vi "uti_IsInSubPanel.vi"(8 "error in (no error)":errorcluster, 11 "UI_Actor in":refnum<class "UI_Actor.lvclass">) -> (0 "error out":errorcluster, 2 "Running in SubPanel?":bool, 3 "UI_Actor out":refnum<class "UI_Actor.lvclass">)   [LabVIEW 2020, in "UI_Actor.lvlib" / "UI_Actor.lvclass"]
uses:
  UI_Actor.lvclass
  UI_Actor.lvclass/UI_Actor.ctl
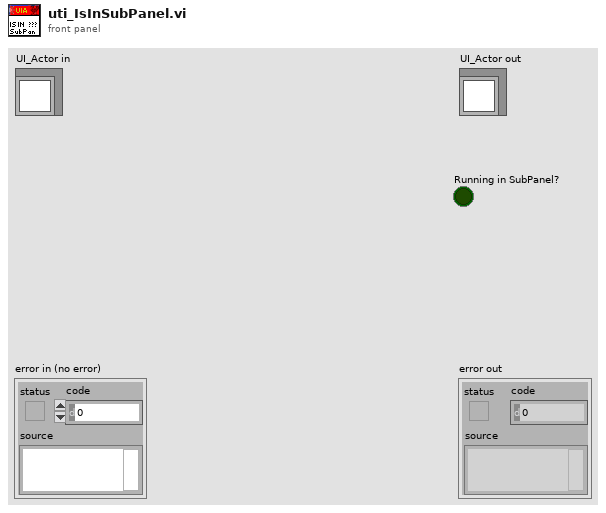
[diagram p1: front panel]
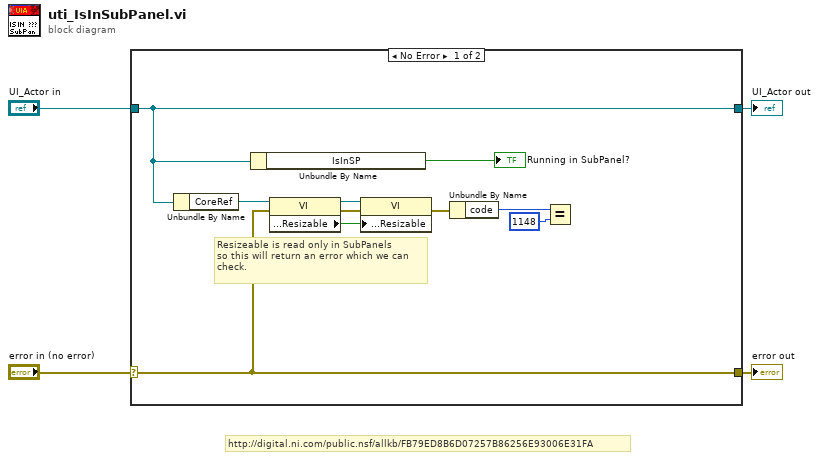
[diagram p0: block diagram]
diagram:
  # "http://digital.ni.com/public.nsf/allkb/FB79ED8B6D07257B86256E93006E31FA"
  n1 = case shown="No Error" "error in (no error)" {
    selector: "error in (no error)" -> [w8 w16]
    tunnel: [w8 w16] -> w3
    tunnel: [w7 w15] -> w1
    tunnel: "UI_Actor in" -> [w7 w15]
    frame No Error {
      # "Resizeable is read only in SubPanels\nso this will return an error which we can\ncheck."
      n2 = Unbundle By Name(w7) -> ("CoreRef"=w9:refnum<vi>)
      n3 = Unbundle By Name(w7) -> ("IsInSP"=→"Running in SubPanel?":bool)
      n4 = property class="VI"(reference=w9, error in=w8) -> (reference out=w11:refnum<vi>, error out=w10:errorcluster, "Front Panel Window:Resizable"=w12:bool)
      n5 = property class="VI"(reference=w11, error in=w10, "Front Panel Window:Resizable"=w12) -> (error out=w13:errorcluster)  [unwired: 1 out]
      n6 = Unbundle By Name(w13) -> ("code"=w6:i32)
      n7 = Equal?(x=w6, y=1148) -> ()  [unwired: 1 out]
    }
    frame Error {
    }
  }
  "error out" <- w3
  "UI_Actor out" <- w1
